vi "ge_Val2String_NChan.vi"(0 "Values":u16[](array[numeric]), 1 "ColType":T1, 2 "DefVal":u16=65535) -> (5 "String and Values":cluster{"String":string, "Value":u16}[](array[cluster]))   [LabVIEW 2012]
uses:
  Custom Ctls Table/ge_ColType.ctl
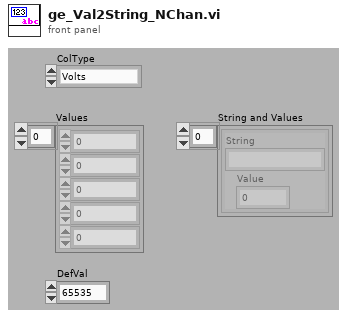
[diagram p1: front panel]
types:
  T1 = typedef "ge_ColType.ctl" = enum16{"Volts", "Amps", "Ohms", "TermCfg", "WireCfg", "Coup", "Slope", "Iex", "CalUnits", "ThrmUnits", "ThrmType", "CJCSrc", "BrdgType", "Strn Mode", "RTDType"}
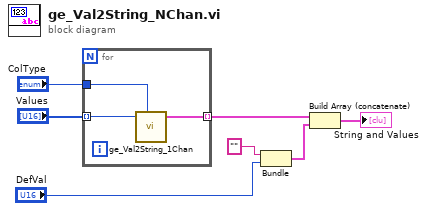
[diagram p0: block diagram]
diagram:
  n1 = for {
    tunnel: "Values" -> [w10] mode=indexing
    tunnel: [w8] -> w6 mode=indexing
    tunnel: "ColType" -> [w9]
    n2 = call "ge_Val2String_1Chan.vi"("Value"=w10, "ColType"=w9) -> ("String and Val"=w8:cluster{"String":string, "Value":u16})  [unwired: 5 in]
  }
  n3 = Bundle("", "DefVal"="DefVal") -> (w2:cluster{string, "DefVal":u16})  [unwired: 1 in]
  n4 = Build Array (concatenate)(w6, w2) -> (→"String and Values":cluster{"String":string, "DefVal":u16}[])
